vi "Broken VI.vi"() -> ()   [LabVIEW 2010]
panel:
  out "Running Result":dbl
  in  "X":dbl
  in  "Calculate":bool
  in  "Action":T1(ring)
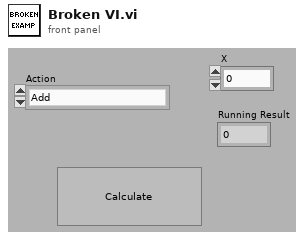
[diagram p1: front panel]
types:
  T1 = enum16{"Add", "Subtract", "Multiply", "Divide", "Set"}
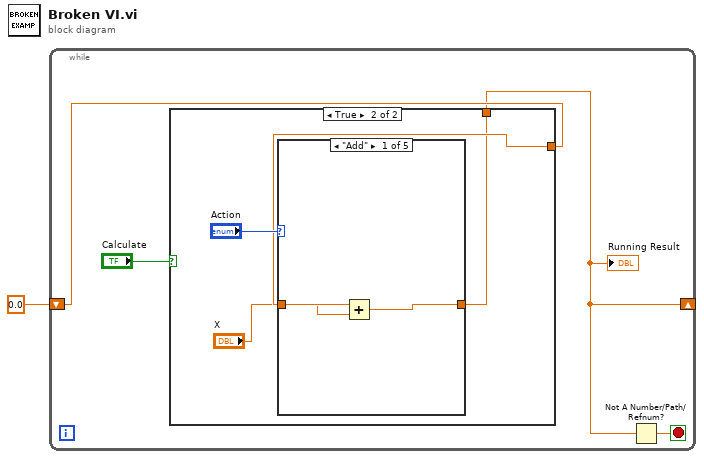
[diagram p0: block diagram]
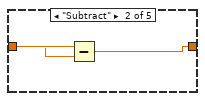
[diagram p3: hidden frame]
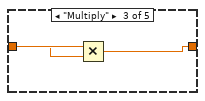
[diagram p4: hidden frame]
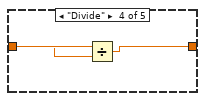
[diagram p5: hidden frame]
diagram:
  n1 = while {
    shift-right: [w2] -> _
    shift-left: 0.0 -> [w4]
    stop <- w2 stop-if-true
    n2 = case shown="True" "Calculate" {
      tunnel: w4 -> [_ w7]
      tunnel: [_ w6] -> w2
      frame False {
      }
      frame True {
        n3 = case shown="\"Add\"" "Action" {
          tunnel: w7 -> [w10 w14 w17 w20 _]
          tunnel: [w11 w12 w15 w18 w21] -> w6
          tunnel: "X" -> [w9 w13 w16 w19 w21]
          frame "Add" {
            n4 = Add(x=w10, y=w9) -> (x+y=w11:dbl)
          }
          frame "Subtract" {
            n5 = Subtract(x=w14, y=w13) -> (x-y=w12:dbl)
          }
          frame "Multiply" {
            n6 = Multiply(x=w17, y=w16) -> (x*y=w15:dbl)
          }
          frame "Divide" {
            n7 = Divide(x=w20, y=w19) -> (x/y=w18:dbl)
          }
          frame "Set", Default {
          }
        }
      }
    }
    "Running Result" <- w2
    n8 = Not A Number/Path/Refnum?(number/path/refnum=w2) -> ()  [unwired: 1 out]
  }
